vi "NewGame.vi"(7 "AboutScreenType (ChildObject)":refnum<class "AboutScreen.lvclass">, 8 "error in (no error)":errorcluster, 11 "FPGA_ref":T1) -> (0 "error out":errorcluster, 3 "AboutScreen out":refnum<class "AboutScreen.lvclass">)   [LabVIEW 2019, in "RT_Game.lvlib" / "AboutScreen.lvclass"]
uses:
  AboutScreen.lvclass
  C:/Users/FreshBob/Dropbox/VIs/myRIO_GameConsole/RT/RT_Game/Game/Game.lvclass
  FPGA_Interface.ctl
  Game/Game.lvclass
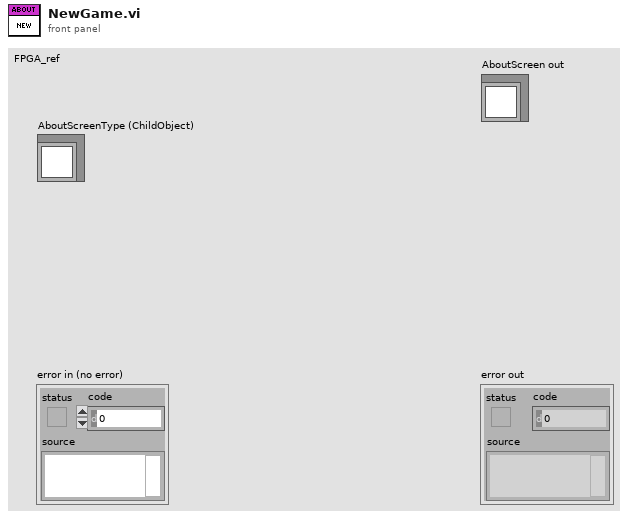
[diagram p1: front panel]
types:
  T1 = typedef "FPGA_Interface.ctl" = refnum<k20>
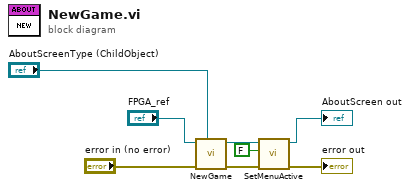
[diagram p0: block diagram]
diagram:
  n1 = call-parent "NewGame.vi"("GameType (ChildObject)"="AboutScreenType (ChildObject)", "error in (no error)"="error in (no error)", "FPGA_ref"="FPGA_ref") -> ("error out"=w8:errorcluster, "Game out"=w3:refnum<class "AboutScreen.lvclass">)  [unwired: 7 in]
  n2 = call "SetMenuActive.vi"("error in (no error)"=w8, "Active?"=FALSE, "Game in"=w3) -> ("error out"=→"error out":errorcluster, "Game out"=→"AboutScreen out":refnum<class "AboutScreen.lvclass">)  [unwired: 7 in]
